vi "SParmCALGUI.vi"(0 "VNA":refnum<visa-resource-name>="GPIB1::16::INSTR", 5 "error in":errorcluster, 7 "Channel":i32=1) -> (8 "CalKit":string[](array[string]), 10 "Conn":string[](array[string]), 12 "Orient":bool, 13 "Exit":bool, 14 "VNA Out":refnum<visa-resource-name>="GPIB1::16::INSTR", 19 "error out":errorcluster={"status"=TRUE, "code"=-1073807346, "source"="VISA Write in SENS_CORR_COLL_GUID_CONN_CAT_ARY.vi->SParmCALGUI.vi"})   [LabVIEW 2018]
uses:
  PNA-X.lvlib
panel:
  in  "Calibration Kit":string(combo)="N4691-60004 ECal"
  out "PORT #":i32=4
  in  "Connector Type":i32(listbox)
  in  "stop":bool
  in  "OK Button":bool
  # "S-Parameter Calibrstion Parameters"
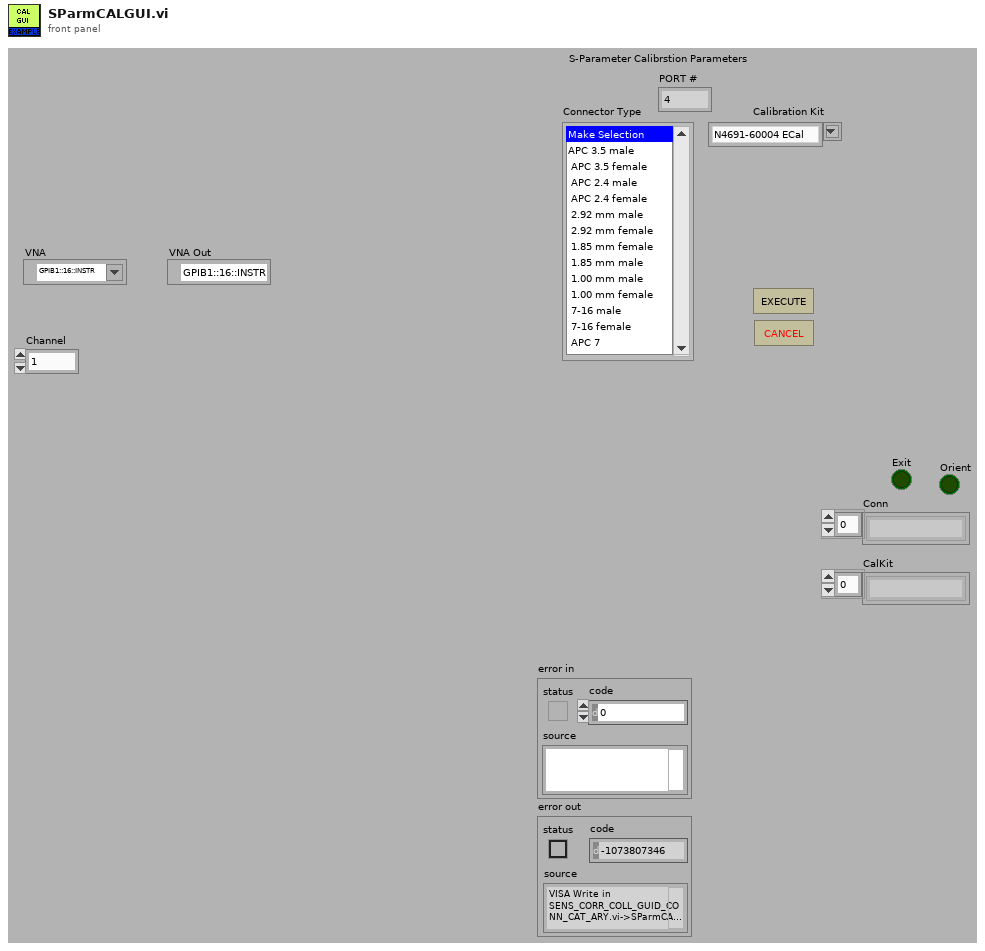
[diagram p1: front panel]
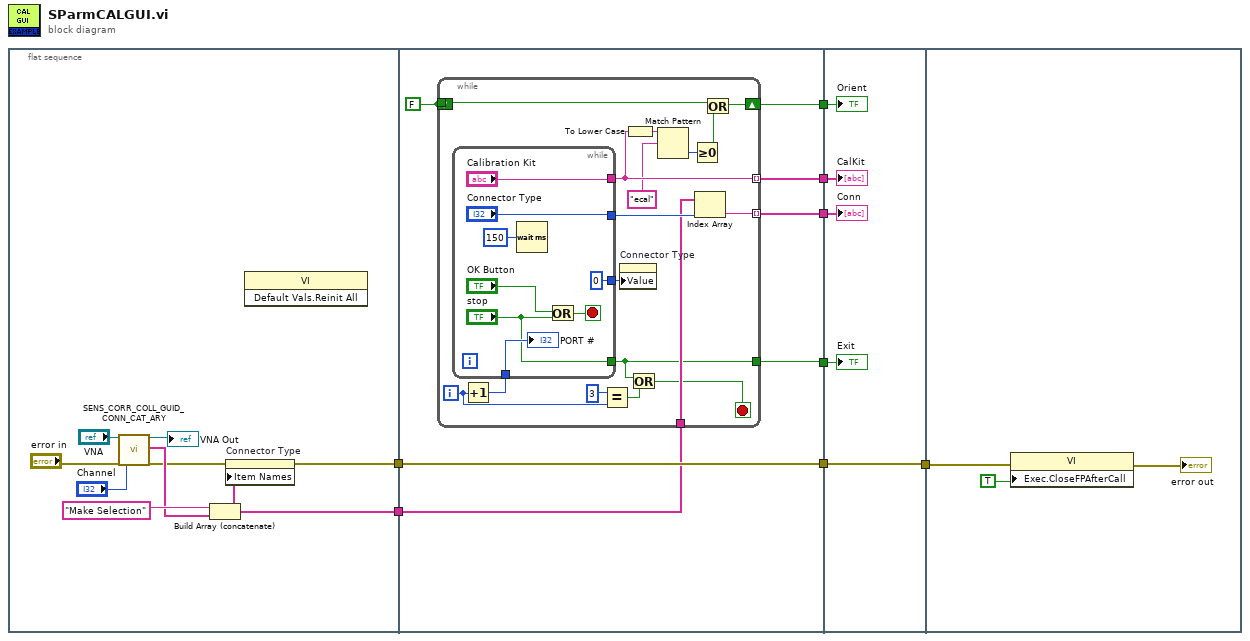
[diagram p0: block diagram]
diagram:
  n1 = flat-sequence {
    tunnel: [w11] -> w7
    tunnel: [w10] -> w6
    tunnel: [w24] -> w8
    tunnel: w7 -> [w24]
    tunnel: w6 -> [w23]
    tunnel: [w22] -> w5
    tunnel: [w21] -> w4
    tunnel: [w19] -> w3
    tunnel: [w18] -> w2
    tunnel: w8 -> [w54]
    tunnel: w5 -> [w51]
    tunnel: w4 -> [w52]
    tunnel: w3 -> [w53]
    tunnel: w2 -> [w50]
    tunnel: [w54] -> w1
    tunnel: w1 -> [w56]
    frame #0 {
      n2 = call "SENS_CORR_COLL_GUID_CONN_CAT_ARY.vi"("VNA"="VNA", "error in"="error in", "Channel"="Channel") -> ("VNA Out"=→"VNA Out":refnum<visa-resource-name>, "ConAry"=w15:string[], "error out"=w12:errorcluster)  [unwired: 14 in]
      n3 = Build Array (concatenate)("Make Selection", w15) -> (w10:string[])
      n4 = property on="Connector Type" class="LstBox (strict)"(error in=w12, "Item Names"=w10) -> (error out=w11:errorcluster)  [unwired: 1 in, 1 out]
      n5 = invoke class="VI" method="Default Vals.Reinit All"() -> ()  [unwired: 3 in, 3 out]
    }
    frame #1 {
      w20 = FALSE
      n6 = while {
        tunnel: [w34] -> w21 mode=indexing
        tunnel: w23 -> [w38]
        tunnel: [w37] -> w22 mode=indexing
        shift-right: [w35] -> w19
        shift-left: w20 -> [_]
        tunnel: w20 -> [w36]
        tunnel: [w25] -> w18
        i -> [w28]
        stop <- w26 stop-if-true
        n7 = Increment(x=w28) -> (x+1=w41:i32)
        n8 = while {
          tunnel: ["Calibration Kit"] -> w34
          tunnel: ["Connector Type"] -> w39
          tunnel: w41 -> [w44]
          tunnel: [0] -> w40
          tunnel: ["stop"] -> w25
          stop <- w49 stop-if-true
          n9 = Wait (ms)(milliseconds to wait=u32 150) -> ()  [unwired: 1 out]
          n10 = Or(x="OK Button", y="stop") -> (x .or. y?=w49:bool)
          "PORT #" <- w44
        }
        n11 = Equal?(x=3, y=w28) -> (x = y?=w27:bool)
        n12 = property on="Connector Type" class="LstBox (strict)"("Value"=w40) -> ()  [unwired: 2 in, 2 out]
        n13 = To Lower Case(string=w34) -> (all lower case string=w33:string)
        n14 = Or(x=w25, y=w27) -> (x .or. y?=w26:bool)
        n15 = Match Pattern(string=w33, regular expression="ecal") -> (offset past match=w31:i32)  [unwired: 1 in, 3 out]
        n16 = Greater Or Equal To 0?(x=w31) -> (x >= 0?=w30:bool)
        n17 = Index Array(array=w38, index=w39) -> (element=w37:string)
        n18 = Or(x=w36, y=w30) -> (x .or. y?=w35:bool)
      }
    }
    frame #2 {
      "Orient" <- w53
      "CalKit" <- w52
      "Conn" <- w51
      "Exit" <- w50
    }
    frame #3 {
      n19 = property class="VI"(error in=w56, "Exec.CloseFPAfterCall"=TRUE ("Execution:Close After Call")) -> (error out=→"error out":errorcluster)  [unwired: 1 in, 1 out]
    }
  }
